vi "SDSETP.vi"(8 "error in (no error)":errorcluster, 10 "Expected response":string, 11 "UI Actor in":refnum<class "UI Actor.lvclass">) -> (0 "error out":errorcluster)   [LabVIEW 2020, in "UI Actor.lvlib" / "UI Actor.lvclass"]
uses:
  UI Actor.lvclass
  UI Actor.lvclass/UI Actor.ctl
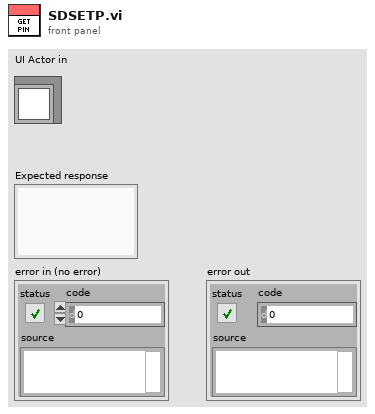
[diagram p1: front panel]
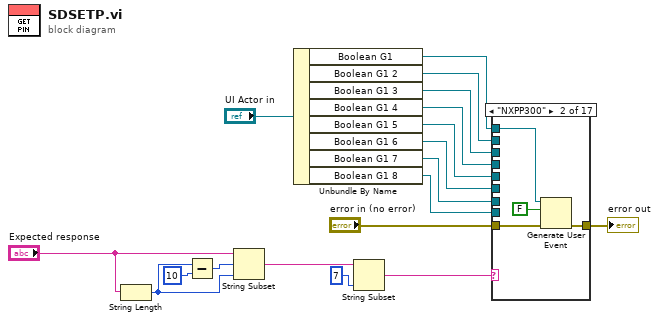
[diagram p0: block diagram]
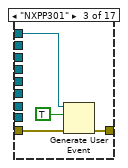
[diagram p3: hidden frame]
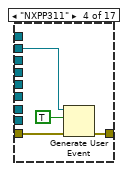
[diagram p4: hidden frame]
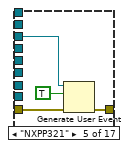
[diagram p5: hidden frame]
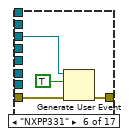
[diagram p6: hidden frame]
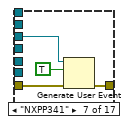
[diagram p7: hidden frame]
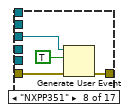
[diagram p8: hidden frame]
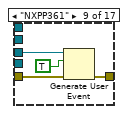
[diagram p9: hidden frame]
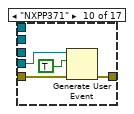
[diagram p10: hidden frame]
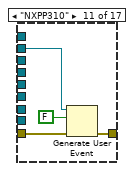
[diagram p11: hidden frame]
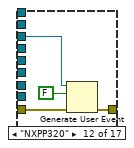
[diagram p12: hidden frame]
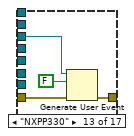
[diagram p13: hidden frame]
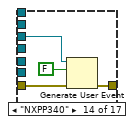
[diagram p14: hidden frame]
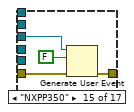
[diagram p15: hidden frame]
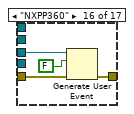
[diagram p16: hidden frame]
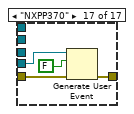
[diagram p17: hidden frame]
diagram:
  n1 = String Length(string="Expected response") -> (length=w4:i32)
  n2 = Subtract(x=w4, y=10) -> (x-y=w6:i32)
  n3 = String Subset(string="Expected response", offset (0)=w6, length (rest)=w4) -> (substring=w3:string)
  n4 = Unbundle By Name("UI Actor in") -> ("Boolean G1"=w18:refnum<user-event>, "Boolean G1 2"=w14:refnum<user-event>, "Boolean G1 3"=w13:refnum<user-event>, "Boolean G1 4"=w12:refnum<user-event>, "Boolean G1 5"=w11:refnum<user-event>, "Boolean G1 6"=w10:refnum<user-event>, "Boolean G1 7"=w9:refnum<user-event>, "Boolean G1 8"=w8:refnum<user-event>)
  n5 = String Subset(string=w3, length (rest)=7 ("length (rest)")) -> (substring=w1:string)  [unwired: 1 in]
  n6 = case shown="\"NXPP300\"" w1 {
    tunnel: w18 -> [_ w21 w25 _ _ _ _ _ _ _ _ _ _ _ _ _ _]
    tunnel: [_ w20 w24 w29 w33 w37 w41 w45 w49 w53 w57 w61 w65 w69 w73 w77 w81] -> w16
    tunnel: "error in (no error)" -> [_ w19 w23 w28 w32 w36 w40 w44 w48 w52 w56 w60 w64 w68 w72 w76 w80]
    tunnel: w14 -> [_ _ _ w27 _ _ _ _ _ _ w55 _ _ _ _ _ _]
    tunnel: w13 -> [_ _ _ _ w31 _ _ _ _ _ _ w59 _ _ _ _ _]
    tunnel: w12 -> [_ _ _ _ _ w35 _ _ _ _ _ _ w63 _ _ _ _]
    tunnel: w11 -> [_ _ _ _ _ _ w39 _ _ _ _ _ _ w67 _ _ _]
    tunnel: w10 -> [_ _ _ _ _ _ _ w43 _ _ _ _ _ _ w71 _ _]
    tunnel: w9 -> [_ _ _ _ _ _ _ _ w47 _ _ _ _ _ _ w75 _]
    tunnel: w8 -> [_ _ _ _ _ _ _ _ _ w51 _ _ _ _ _ _ w79]
    frame "False", Default {
    }
    frame "NXPP300" {
      n7 = Generate User Event(user event=w21, event data cluster=FALSE ("event data"), error in=w19) -> (error out=w20:errorcluster)  [unwired: 1 in, 1 out]
    }
    frame "NXPP301" {
      n8 = Generate User Event(user event=w25, event data cluster=TRUE ("event data"), error in=w23) -> (error out=w24:errorcluster)  [unwired: 1 in, 1 out]
    }
    frame "NXPP311" {
      n9 = Generate User Event(user event=w27, event data cluster=TRUE ("event data"), error in=w28) -> (error out=w29:errorcluster)  [unwired: 1 in, 1 out]
    }
    frame "NXPP321" {
      n10 = Generate User Event(user event=w31, event data cluster=TRUE ("event data"), error in=w32) -> (error out=w33:errorcluster)  [unwired: 1 in, 1 out]
    }
    frame "NXPP331" {
      n11 = Generate User Event(user event=w35, event data cluster=TRUE ("event data"), error in=w36) -> (error out=w37:errorcluster)  [unwired: 1 in, 1 out]
    }
    frame "NXPP341" {
      n12 = Generate User Event(user event=w39, event data cluster=TRUE ("event data"), error in=w40) -> (error out=w41:errorcluster)  [unwired: 1 in, 1 out]
    }
    frame "NXPP351" {
      n13 = Generate User Event(user event=w43, event data cluster=TRUE ("event data"), error in=w44) -> (error out=w45:errorcluster)  [unwired: 1 in, 1 out]
    }
    frame "NXPP361" {
      n14 = Generate User Event(user event=w47, event data cluster=TRUE ("event data"), error in=w48) -> (error out=w49:errorcluster)  [unwired: 1 in, 1 out]
    }
    frame "NXPP371" {
      n15 = Generate User Event(user event=w51, event data cluster=TRUE ("event data"), error in=w52) -> (error out=w53:errorcluster)  [unwired: 1 in, 1 out]
    }
    frame "NXPP310" {
      n16 = Generate User Event(user event=w55, event data cluster=FALSE ("event data"), error in=w56) -> (error out=w57:errorcluster)  [unwired: 1 in, 1 out]
    }
    frame "NXPP320" {
      n17 = Generate User Event(user event=w59, event data cluster=FALSE ("event data"), error in=w60) -> (error out=w61:errorcluster)  [unwired: 1 in, 1 out]
    }
    frame "NXPP330" {
      n18 = Generate User Event(user event=w63, event data cluster=FALSE ("event data"), error in=w64) -> (error out=w65:errorcluster)  [unwired: 1 in, 1 out]
    }
    frame "NXPP340" {
      n19 = Generate User Event(user event=w67, event data cluster=FALSE ("event data"), error in=w68) -> (error out=w69:errorcluster)  [unwired: 1 in, 1 out]
    }
    frame "NXPP350" {
      n20 = Generate User Event(user event=w71, event data cluster=FALSE ("event data"), error in=w72) -> (error out=w73:errorcluster)  [unwired: 1 in, 1 out]
    }
    frame "NXPP360" {
      n21 = Generate User Event(user event=w75, event data cluster=FALSE ("event data"), error in=w76) -> (error out=w77:errorcluster)  [unwired: 1 in, 1 out]
    }
    frame "NXPP370" {
      n22 = Generate User Event(user event=w79, event data cluster=FALSE ("event data"), error in=w80) -> (error out=w81:errorcluster)  [unwired: 1 in, 1 out]
    }
  }
  "error out" <- w16
